vi "PH_Stepmotor_BaseClass.PC set Target.vi"(0 "VI in":refnum<vi>, 2 "axis":i32=-1, 3 "Targetposition to set":i32, 5 "error in (no error)":errorcluster) -> (14 "VI out":refnum<vi>, 19 "error out":errorcluster)   [LabVIEW 2014, in "PH_Stepmotor_BaseClass.lvlib"]
doc: "This VI sets Values to own attributes."
uses:
  PH_Stepmotor_BaseClass.lvlib
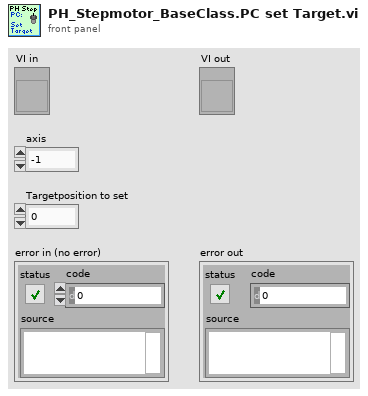
[diagram p1: front panel]
types:
  T1 = typedef "PH_Stepmotor_BaseClass.lvlib/PH_Stepmotor_BaseClass.Axis Attributes.ctl" = cluster{"Settings":T2, "Endswitch?":bool, "DIM Service IDs":T4, "Activity":T5, "Configured?":bool, "Position":cluster{"Current":i32, "Target":i32}, "Position to set":cluster{"New?":bool, "Wanted":i32}, "Stop?":bool, "Reset?":bool, "Move?":bool, "Nothing connected?":bool}
  T2 = typedef "PH_Stepmotor_BaseClass.lvlib/PH_Stepmotor_BaseClass.Axis Settings.ctl" = cluster{"Sign change":bool, "Width":dbl, "Calibration":dbl, "Unit":string, "Motor Type":T3, "Unit Width":string, "Unit CF":string}
  T3 = typedef "PH_Stepmotor_BaseClass.lvlib/PH_Stepmotor_BaseClass.Motor Type.ctl" = enum16{"Unspecific", "OWIS 49.120.2633", "OWIS 49.060.1033", "OWIS 43.040.2558", "Diamond Motion 2200 series", "OWIS 49.120.266B.MV6", "Calorimeter", "Linear Stage 1", "MICOS VT-80", "MICOS VT-80 S", "Standa Rotstage nt0.95A", "PUF RA 320.200", "PUF RA 800.200", "PUF RA 800.400", "PUF RA 400.50", "1324.nn.800.50", "1324.n9c.800.50", "1324.nn.320.200", "1324.nn.400.200", "1324.nn.800.200", "1324.nn.400.50", "1324.8c9c.800.50", "1324.8c9c.400.200"}
  T4 = typedef "PH_Stepmotor_BaseClass.lvlib/PH_Stepmotor_BaseClass.Axis DIM Service IDs.ctl" = cluster{"Settings":i32, "Information":i32}
  T5 = typedef "PH_Stepmotor_BaseClass.lvlib/PH_Stepmotor_BaseClass.Axis Activity.ctl" = enum16{"No Information", "stopped", "running", "Failure", "Alarm", "stopped at backward ES", "stopped at foreward ES"}
  T6 = typedef "PH_Stepmotor_BaseClass.lvlib/PH_Stepmotor_BaseClass.i attribute.ctl" = cluster{"Device Error":errorcluster, "Axes PSDB Thread":cluster{"Ref":refnum<vi>, "Q-Ref":refnum<queue>, "Data Status":T7}, "Axes":T1[], "Axes PSDB Infos":cluster{"GUI Name":string, "PSDB Instance ID":i32, "PSDB Status Service ID":i32, "Axis":i32, "Class":string}[], "GUI Refs":T8}
  T7 = typedef "PH_PSDBWriter.lvlib/PH_PSDBWriter.Data Status.ctl" = i16
  T8 = typedef "PH_Stepmotor_BaseClass.lvlib/PH_Stepmotor_BaseClass.GUI Refs.ctl" = cluster{"Axes Configuration":refnum<vi>, "Device Error":refnum<vi>, "Axes PSDB Infos":refnum<vi>}
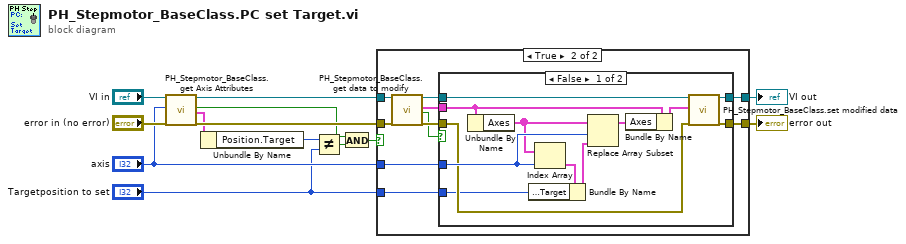
[diagram p0: block diagram]
diagram:
  n1 = call "PH_Stepmotor_BaseClass.get Axis Attributes.vi"("VI in"="VI in", "Axis"="axis", "error in (no error)"="error in (no error)") -> ("VI out"=w8:refnum<vi>, "Axis found?"=w3:bool, "Axis Attributes"=w6:T1, "error out"=w10:errorcluster)  [unwired: 13 in]
  n2 = Unbundle By Name(w6) -> ("Position.Target"=w5:i32)
  n3 = Not Equal?(x=w5, y="Targetposition to set") -> (x != y?=w1:bool)
  n4 = And(x=w3, y=w1) -> (x .and. y?=w2:bool)
  n5 = case shown="True" w2 {
    tunnel: [w14 w25] -> w12
    tunnel: [w15 w24] -> w11
    tunnel: w10 -> [w14 w19]
    tunnel: w8 -> [w15 w18]
    tunnel: "axis" -> [_ w17]
    tunnel: "Targetposition to set" -> [_ w16]
    frame False {
    }
    frame True {
      n6 = call "PH_Stepmotor_BaseClass.get data to modify.vi"("i ref in"=w18, "error in (no error)"=w19) -> ("i ref out"=w22:refnum<vi>, "i attribute"=w23:T6, "timed out"=w20:bool, "error out"=w21:errorcluster)  [unwired: 14 in]
      n7 = case shown="False" w20 {
        tunnel: [w37 w39] -> w25
        tunnel: w21 -> [w27 w39]
        tunnel: [w36 w38] -> w24
        tunnel: w22 -> [w32 w38]
        tunnel: w23 -> [w35 _]
        tunnel: w17 -> [w31 _]
        tunnel: w16 -> [w26 _]
        frame False {
          n8 = Unbundle By Name(w35) -> ("Axes"=w29:T1[])
          n9 = Index Array(array=w29, index=w31) -> (element=w28:T1)
          n10 = Bundle By Name(cluster=w28, "Position.Target"=w26) -> (w30:T1)
          n11 = Replace Array Subset(array=w29, new element=w30, index=w31) -> (w33:T1[])
          n12 = Bundle By Name(cluster=w35, "Axes"=w33) -> (w34:T6)
          n13 = call "PH_Stepmotor_BaseClass.set modified data.vi"("i ref in"=w32, "i attribute"=w34, "error in (no error)"=w27) -> ("i ref out"=w36:refnum<vi>, "error out"=w37:errorcluster)  [unwired: 15 in]
        }
        frame True {
          (unwired) TRUE
        }
      }
    }
  }
  "error out" <- w12
  "VI out" <- w11
